vi "00_SpectrometerTest.vi"() -> ()   [LabVIEW 2018]
uses:
  <instrlib>/Classes/CCD/Avantes/Avantes.lvclass
panel:
  in  "Exposure Time 2":dbl[unit]
  in  "Frames 2":i32 min=1
  out "Data":T1(array[cluster])
  out "Data Raw":T1(array[cluster])
  out "Darkspec":T1(array[cluster])
  out "Time":dbl[](array[numeric])
  out "lambda":dbl[unit][](array[numeric])
  out "Frames":i32=-5000
  out "Frame Rate":dbl[unit]
  out "Exposure Time":dbl[unit]
  out "Exposure per Frame":i32=-5000
  out "Is Init?":bool
  out "error out":errorcluster
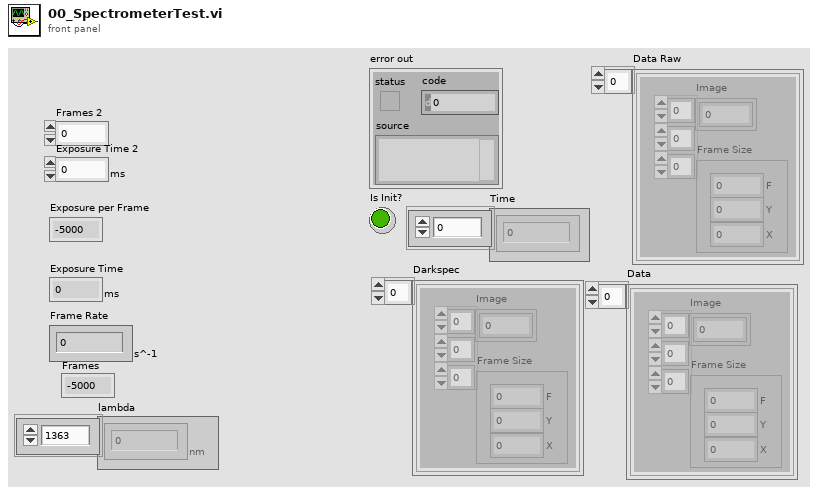
[diagram p1: front panel]
types:
  T1 = cluster{"Image":dbl[][][], "Frame Size":cluster{"F":i32, "Y":i32, "X":i32}}[]
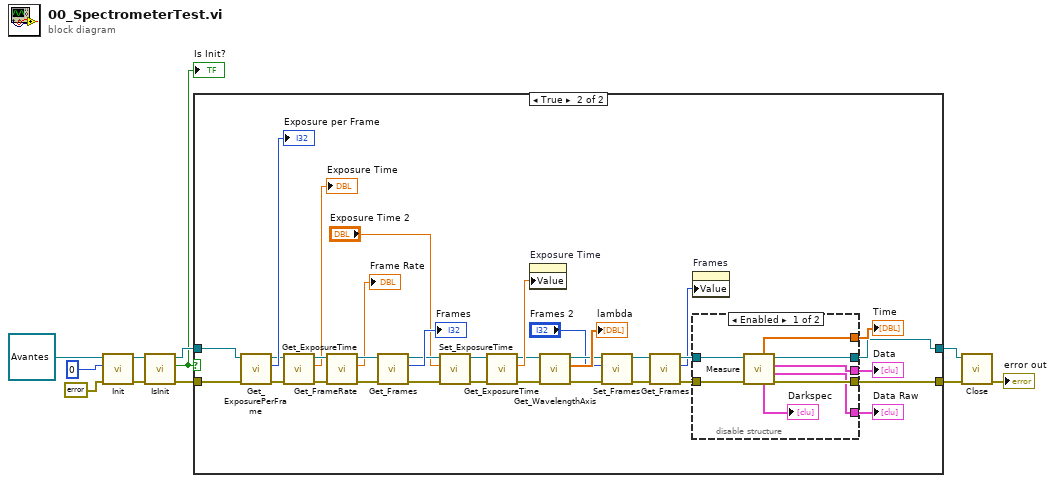
[diagram p0: block diagram]
diagram:
  n1 = call-dynamic "Init.vi"("error in (no error)"=errorcluster {"status"=FALSE, "code"=0, "source"=""}, "Variant"=0, "Avantes in"=refnum<class "Avantes.lvclass"> refnum ("Avantes.lvclass")) -> ("error out"=w7:errorcluster, "Avantes out"=w8:refnum<class "Avantes.lvclass">)  [unwired: 7 in]
  n2 = call-dynamic "IsInit.vi"("error in (no error)"=w7, "Avantes in"=w8) -> ("error out"=w4:errorcluster, "Is Init?"=w1:bool, "Avantes out"=w5:refnum<class "Avantes.lvclass">)  [unwired: 7 in]
  "Is Init?" <- w1
  n3 = case shown="True" w1 {
    tunnel: w5 -> [w13 w47]
    tunnel: w4 -> [w12 w46]
    tunnel: [w13 w33] -> w3
    tunnel: [w12 w32] -> w2
    frame False {
    }
    frame True {
      n4 = call-dynamic "Get_ExposurePerFrame.vi"("error in (no error)"=w46, "Avantes in"=w47) -> ("error out"=w43:errorcluster, "Exposure per Frame"=→"Exposure per Frame":i32, "Avantes out"=w44:refnum<class "Avantes.lvclass">)  [unwired: 7 in]
      n5 = call-dynamic "Get_ExposureTime.vi"("error in (no error)"=w43, "Avantes in"=w44) -> ("error out"=w41:errorcluster, "Exposure Time"=→"Exposure Time":dbl[unit], "Avantes out"=w42:refnum<class "Avantes.lvclass">)  [unwired: 7 in]
      n6 = call-dynamic "Get_FrameRate.vi"("error in (no error)"=w41, "Avantes in"=w42) -> ("error out"=w38:errorcluster, "Frame Rate"=→"Frame Rate":dbl[unit], "Avantes out"=w39:refnum<class "Avantes.lvclass">)  [unwired: 7 in]
      n7 = call-dynamic "Get_Frames.vi"("error in (no error)"=w38, "Avantes in"=w39) -> ("error out"=w20:errorcluster, "Frames"=→"Frames":i32, "Avantes out"=w21:refnum<class "Avantes.lvclass">)  [unwired: 7 in]
      n8 = call-dynamic "Set_ExposureTime.vi"("error in (no error)"=w20, "Exposure Time"="Exposure Time 2", "Avantes in"=w21) -> ("error out"=w17:errorcluster, "Avantes out"=w18:refnum<class "Avantes.lvclass">)  [unwired: 7 in]
      n9 = call-dynamic "Get_ExposureTime.vi"("error in (no error)"=w17, "Avantes in"=w18) -> ("error out"=w15:errorcluster, "Exposure Time"=w16:dbl[unit], "Avantes out"=w14:refnum<class "Avantes.lvclass">)  [unwired: 7 in]
      n10 = property on="Exposure Time" class="DigNum (strict)"("Value"=w16) -> ()  [unwired: 2 in, 2 out]
      n11 = call-dynamic "Get_WavelengthAxis.vi"("error in (no error)"=w15, "Avantes in"=w14) -> ("error out"=w28:errorcluster, "lambda"=→"lambda":dbl[unit][], "Avantes out"=w29:refnum<class "Avantes.lvclass">)  [unwired: 7 in]
      n12 = call-dynamic "Set_Frames.vi"("error in (no error)"=w28, "Frames"="Frames 2", "Avantes in"=w29) -> ("error out"=w25:errorcluster, "Avantes out"=w26:refnum<class "Avantes.lvclass">)  [unwired: 7 in]
      n13 = call-dynamic "Get_Frames.vi"("error in (no error)"=w25, "Avantes in"=w26) -> ("error out"=w23:errorcluster, "Frames"=w22:i32, "Avantes out"=w24:refnum<class "Avantes.lvclass">)  [unwired: 7 in]
      n14 = property on="Frames" class="DigNum (strict)"("Value"=w22) -> ()  [unwired: 2 in, 2 out]
      n15 = disable-structure shown="Enabled" {
        disable-tunnel: [w55 _] -> w34
        disable-tunnel: [w54 w57] -> w33
        disable-tunnel: [w53 w56] -> w32
        disable-tunnel: [w51 _] -> w31
        disable-tunnel: [w50 _] -> w30
        disable-tunnel: w24 -> [w49 w57]
        disable-tunnel: w23 -> [w48 w56]
        frame Enabled {
          n16 = call-dynamic "Measure.vi"("error in (no error)"=w48, "Avantes in"=w49) -> ("error out"=w53:errorcluster, "Data Raw"=w51:T1, "Data"=w50:T1, "Avantes out"=w54:refnum<class "Avantes.lvclass">, "Darkspec"=→"Darkspec":T1, "Time"=w55:dbl[])  [unwired: 4 in]
        }
        frame Disabled {
        }
      }
      "Time" <- w34
      "Data Raw" <- w31
      "Data" <- w30
    }
  }
  n17 = call-dynamic "Close.vi"("error in (no error)"=w2, "Avantes in"=w3) -> ("error out"=→"error out":errorcluster)  [unwired: 8 in, 1 out]
